vi "Read Joystick.vi"(8 "Joystick Deadbanded Value (default of 0.1)":dbl, 11 "Joystick L 1 DevRef":T1) -> (1 "Joystick R 2 X Axis":dbl, 2 "Joystick L 1 Y Axis":dbl, 3 "Joystick L 1 X Axis":dbl)   [LabVIEW 2013]
uses:
  <vilib>/Rock Robotics/WPI/Joystick/WPI_JoystickDevRef.ctl
  <vilib>/Rock Robotics/WPI/Joystick/WPI_JoystickDeviceEnum.ctl
  Begin/Global Variables.vi
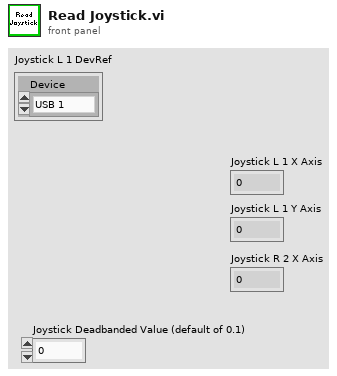
[diagram p1: front panel]
types:
  T1 = typedef "WPI_JoystickDevRef.ctl" = cluster{"Device":T2}
  T2 = typedef "WPI_JoystickDeviceEnum.ctl" = enum16{"USB 1", "USB 2", "USB 3", "USB 4", "Kinect 1", "Kinect 2"}
  T3 = typedef "WPI_JoystickButtonState.ctl" = cluster{"Button 1":bool, "Button 2":bool, "Button 3":bool, "Button 4":bool, "Button 5":bool, "Button 6":bool, "Button 7":bool, "Button 8":bool, "Button 9":bool, "Button 10":bool, "Button 11":bool, "Button 12":bool}
  T4 = cluster{"axis 1 (x)":dbl, "axis 2 (y)":dbl, "axis 3 (throttle)":dbl, "axis 4":dbl, "axis 5":dbl, "axis 6":dbl}
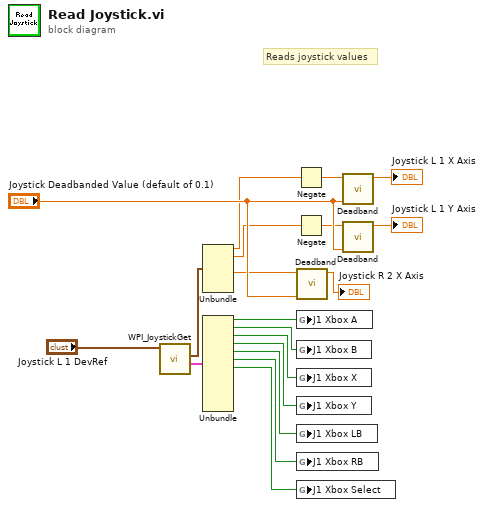
[diagram p0: block diagram]
diagram:
  # "Reads joystick values"
  n1 = call <vilib>:"WPI_JoystickGet.vi"("JoystickDevRef"="Joystick L 1 DevRef") -> ("Buttons"=w19:T3, "Axes"=w18:T4)  [unwired: 4 in, 1 out]
  n2 = Unbundle(w18) -> ("axis 1 (x)"=w7:dbl, "axis 2 (y)"=w12:dbl, "axis 4"=w3:dbl)  [unwired: 3 out]
  n3 = Unbundle(w19) -> ("Button 1"=w1:bool, "Button 2"=w4:bool, "Button 3"=w9:bool, "Button 4"=w5:bool, "Button 5"=w10:bool, "Button 6"=w11:bool, "Button 7"=w2:bool)  [unwired: 5 out]
  n4 = Negate(x=w7) -> (-x=w8:dbl)
  n5 = Negate(x=w12) -> (-x=w6:dbl)
  n6 = call "Deadband.vi"("Value to Deadband (default of 0.1)"="Joystick Deadbanded Value (default of 0.1)", "Value"=w3) -> ("Deadbanded Value"=→"Joystick R 2 X Axis":dbl)  [unwired: 9 in]
  n7 = global write "Global Variables.vi" "J1 Xbox A"(w1) -> ()
  n8 = global write "Global Variables.vi" "J1 Xbox B"(w4) -> ()
  n9 = global write "Global Variables.vi" "J1 Xbox X"(w9) -> ()
  n10 = global write "Global Variables.vi" "J1 Xbox Y"(w5) -> ()
  n11 = global write "Global Variables.vi" "J1 Xbox LB"(w10) -> ()
  n12 = global write "Global Variables.vi" "J1 Xbox RB"(w11) -> ()
  n13 = global write "Global Variables.vi" "J1 Xbox Select"(w2) -> ()
  n14 = call "Deadband.vi"("Value to Deadband (default of 0.1)"="Joystick Deadbanded Value (default of 0.1)", "Value"=w8) -> ("Deadbanded Value"=→"Joystick L 1 X Axis":dbl)  [unwired: 9 in]
  n15 = call "Deadband.vi"("Value to Deadband (default of 0.1)"="Joystick Deadbanded Value (default of 0.1)", "Value"=w6) -> ("Deadbanded Value"=→"Joystick L 1 Y Axis":dbl)  [unwired: 9 in]
